vi "UIbench.vi"() -> ()   [LabVIEW 2017]
panel:
  in  "Skip tabbing":bool=TRUE
  in  "Tab Control":enum32{"Page 1", "Page 2", "Page 3"}(tab)
  in  "Knob":dbl(knob) scale=0.0..10.0
  in  "Stop":bool=TRUE
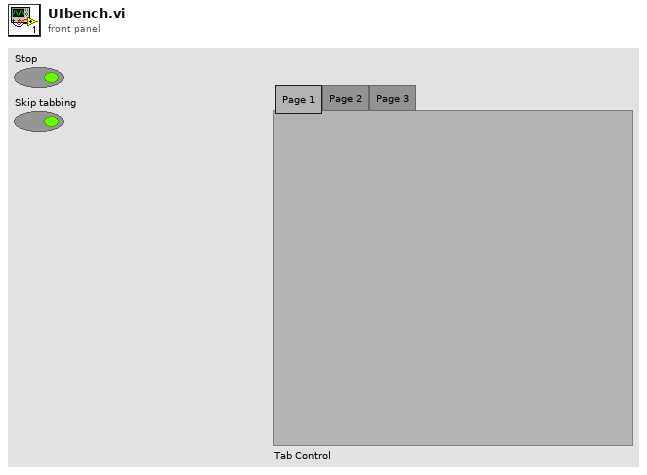
[diagram p1: front panel]
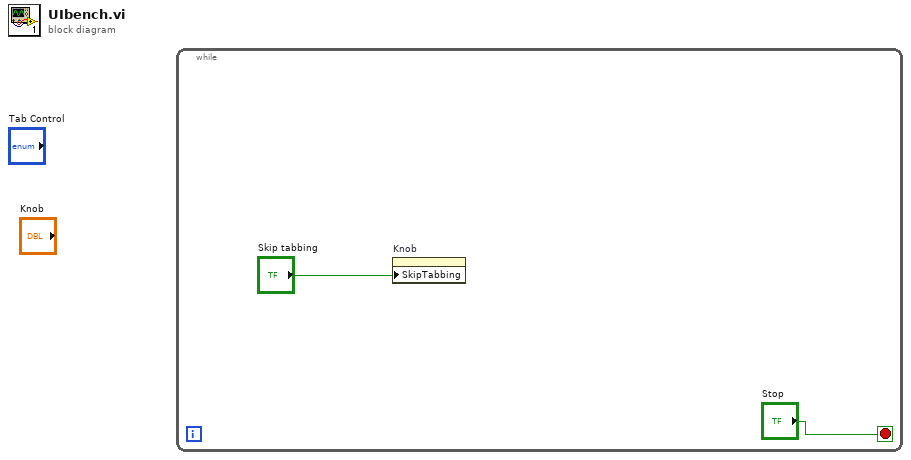
[diagram p0: block diagram]
diagram:
  n1 = while {
    stop <- "Stop" stop-if-true
    n2 = property on="Knob" class="Knob (strict)"("SkipTabbing"="Skip tabbing") -> ()  [unwired: 2 in, 2 out]
  }
